vi "jsonInsertI64.vi"(8 "error in (no error)":errorcluster, 9 "value":i64, 10 "path":string, 11 "d in":i64) -> (0 "error out":errorcluster, 1 "replaced?":bool, 3 "d out":i64)   [LabVIEW 2015, in "JSON Document.lvclass"]
uses:
  API/JSON Document Class/JSON Document.lvclass
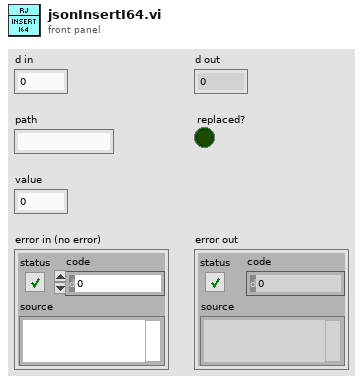
[diagram p1: front panel]
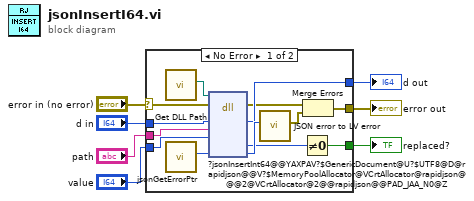
[diagram p0: block diagram]
diagram:
  n1 = case shown="No Error" "error in (no error)" {
    selector: "error in (no error)" -> [w13 w22]
    tunnel: [w10 w22] -> w7
    tunnel: "value" -> [w17 _]
    tunnel: "d in" -> [w16 w21]
    tunnel: "path" -> [w15 _]
    tunnel: [w14 w21] -> w2
    tunnel: [w8 _] -> w1
    frame No Error {
      n2 = call "Get DLL Path.vi"() -> ("Path"=w20:path)  [unwired: 11 in]
      n3 = call "jsonGetErrorPtr.vi"() -> ("return type"=w18:i64)  [unwired: 10 in, 1 out]
      n4 = dll-call lib="C:/Users/tblair/Documents/Git Projects/rapidjson-for-LabVIEW/lvrjs/Debug/lvrjs.dll" fn="?jsonInsertInt64@@YAXPAV?$GenericDocument@U?$UTF8@D@rapidjson@@V?$MemoryPoolAllocator@VCrtAllocator@rapidjson@@@2@VCrtAllocator@2@@rapidjson@@PAD_JAA_N0@Z"(path in=w20, error in=w13, "d"=w16, "path"=w15, "value"=w17, "jsonError"=w18) -> (error out=w12:errorcluster, "d"=w14:i64, "replaced"=w9:i32, "jsonError"=w19:i64)  [unwired: 5 in, 1 out]
      n5 = call "JSON error to LV error.vi"("jsonError"=w19) -> ("error out"=w11:errorcluster)  [unwired: 10 in]
      n6 = Not Equal To 0?(x=w9) -> (x != 0?=w8:bool)
      n7 = Merge Errors(w12, w11) -> (w10:errorcluster)
    }
    frame Error {
    }
  }
  "error out" <- w7
  "d out" <- w2
  "replaced?" <- w1
